vi "Exclude Empty Buffer error (SubVI).vi"(8 "error in":errorcluster) -> (0 "error out":errorcluster)   [LabVIEW 2023, in "PCAN API.lvlib"]
uses:
  PCAN API.lvlib
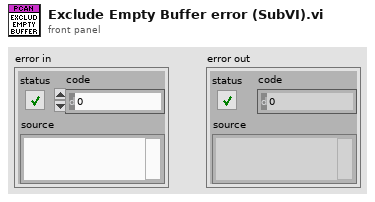
[diagram p1: front panel]
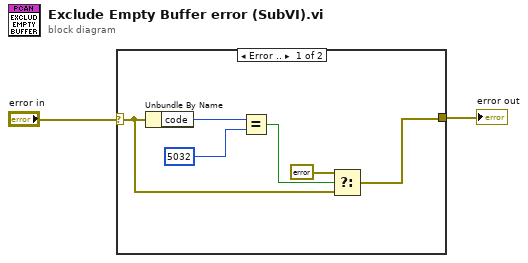
[diagram p0: block diagram]
diagram:
  n1 = case shown="Error .." "error in" {
    selector: "error in" -> [w5 w9]
    tunnel: [w3 w9] -> w1
    frame Error {
      n2 = Unbundle By Name(w5) -> ("code"=w8:i32)
      n3 = Equal?(x=w8, y=5032) -> (x = y?=w6:bool)
      n4 = Select(t=errorcluster {"status"=FALSE, "code"=0, "source"=""}, s=w6, f=w5) -> (s? t:f=w3:errorcluster)
    }
    frame No Error {
    }
  }
  "error out" <- w1
